vi "Main.vi"() -> ()   [LabVIEW 2010]
uses:
  GlobalVar.vi
  <vilib>/Instr/_visa.llb/VISA Configure Serial Port (Instr).vi
panel:
  out "Enum":T1(ring)
  out "error":errorcluster
  out "error Connexion":errorcluster
  out "Stop main loop":bool
  in  "stop":bool
  in  "Tab Control":T2(tab)
  out "Comm_LEDTest":bool
  out "Comm_Reception":string caption="Reception"
  in  "Comm_TestConnection":bool
  in  "baud rate":u32=9600
  in  "VISA resource name":refnum<visa-resource-name>="COM1"
  in  "timeout (10sec)":u32=10000
  out "Erreur courant":bool
  in  "Intensity (A)":string[][](array[string])
  in  "Motor right Torque (N.m)":string[][](array[string])
  out "Motor left Torque (N.m)":string[][](array[string])
  out "Batterie":string[][](array[string])
  out "Guidon":string[][](array[string])
  out "Gyroscope":string[][](array[string])
  out "AccZ":string[][](array[string])
  out "AccX":string[][](array[string])
  out "Acceleration":string[][](array[string])
  out "Velocity motor right":string[][](array[string])
  out "Velocity motor left":string[][](array[string])
  out "Angle Out of range":string[][](array[string])
  out "Speed saturation":string[][](array[string])
  out "Distance parcourue":string[][](array[string])
  out "Angle":string[][](array[string])
  out "XY Graph 2":cluster{dbl, dbl}[](graph)
  out "XY Graph":cluster{dbl, dbl}[](graph)
  in  "Time 3":dbl
  in  "Time 2":dbl
  in  "Time":dbl
  in  "Frequency 3":dbl
  out "Combo Box 3":string(combo)
  in  "Frequency 2":dbl
  out "Combo Box 2":string(combo)
  in  "Ana_SendAnalysis":bool
  in  "Frequency":dbl
  in  "Combo Box":string(combo)
  out "XY Graph 3":cluster{dbl, dbl}[](graph)
  in  "VelocitySaturation":dbl
  in  "Set velocity saturation":bool
  out "Chaîne 2":string
  out "Chaîne":string
  in  "Ready ?":bool
  in  "Current state ?":bool
  in  "Re Start system":bool
  in  "STOP system":bool
  out "tCoef Kalman":dbl
  in  "Bouton OK 11":bool
  in  "Bouton OK 10":bool
  in  "Coef Kalman":dbl
  in  "Bouton OK 9":bool
  in  "Coef System Acc":dbl
  out "tCoef DIR":dbl
  in  "Bouton OK 8":bool
  in  "Coef DIR":dbl
  in  "Bouton OK 7":bool
  out "tD":dbl
  out "tI":dbl
  out "tK":dbl
  in  "Bouton OK 6":bool
  in  "Bouton OK 5":bool
  in  "Bouton OK 4":bool
  in  "Bouton OK 3":bool
  in  "Bouton OK 2":bool
  in  "Bouton OK":bool
  in  "D":dbl
  in  "I":dbl
  in  "K":dbl
  in  "OK Button":bool
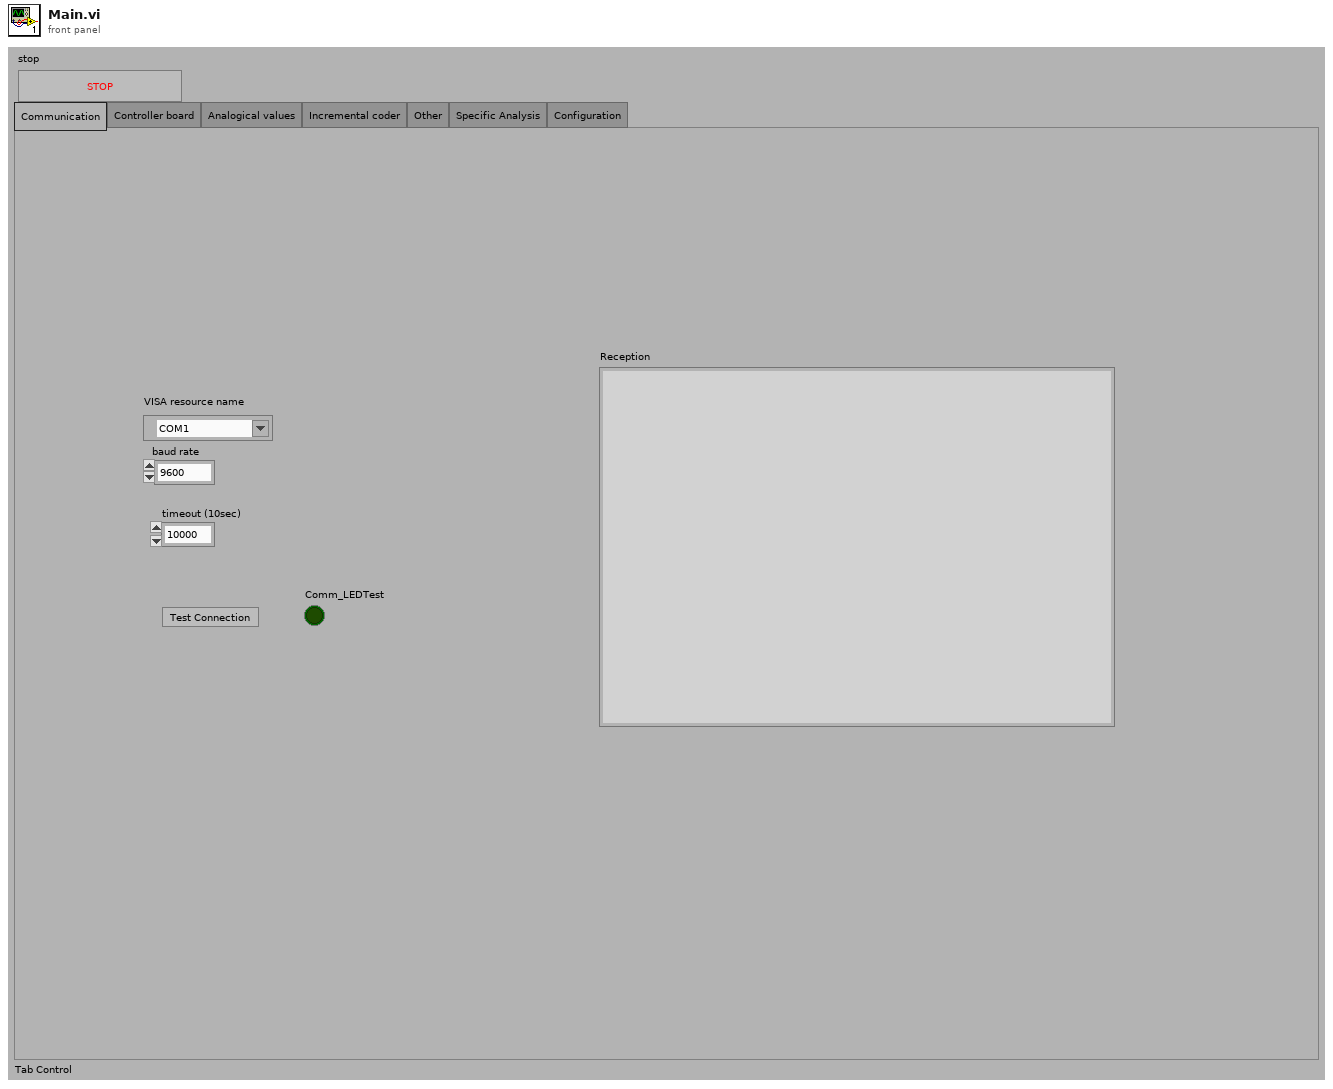
[diagram p1: front panel]
types:
  T1 = enum16{"SendAnalysis", "TestConnection", "Waiting"}
  T2 = enum32{"Communication", "Controller board", "Analogical values", "Incremental coder", "Other", "Specific Analysis", "Configuration"}
  T3 = enum8{"Enabled", "Disabled", "Disabled and Grayed Out"}
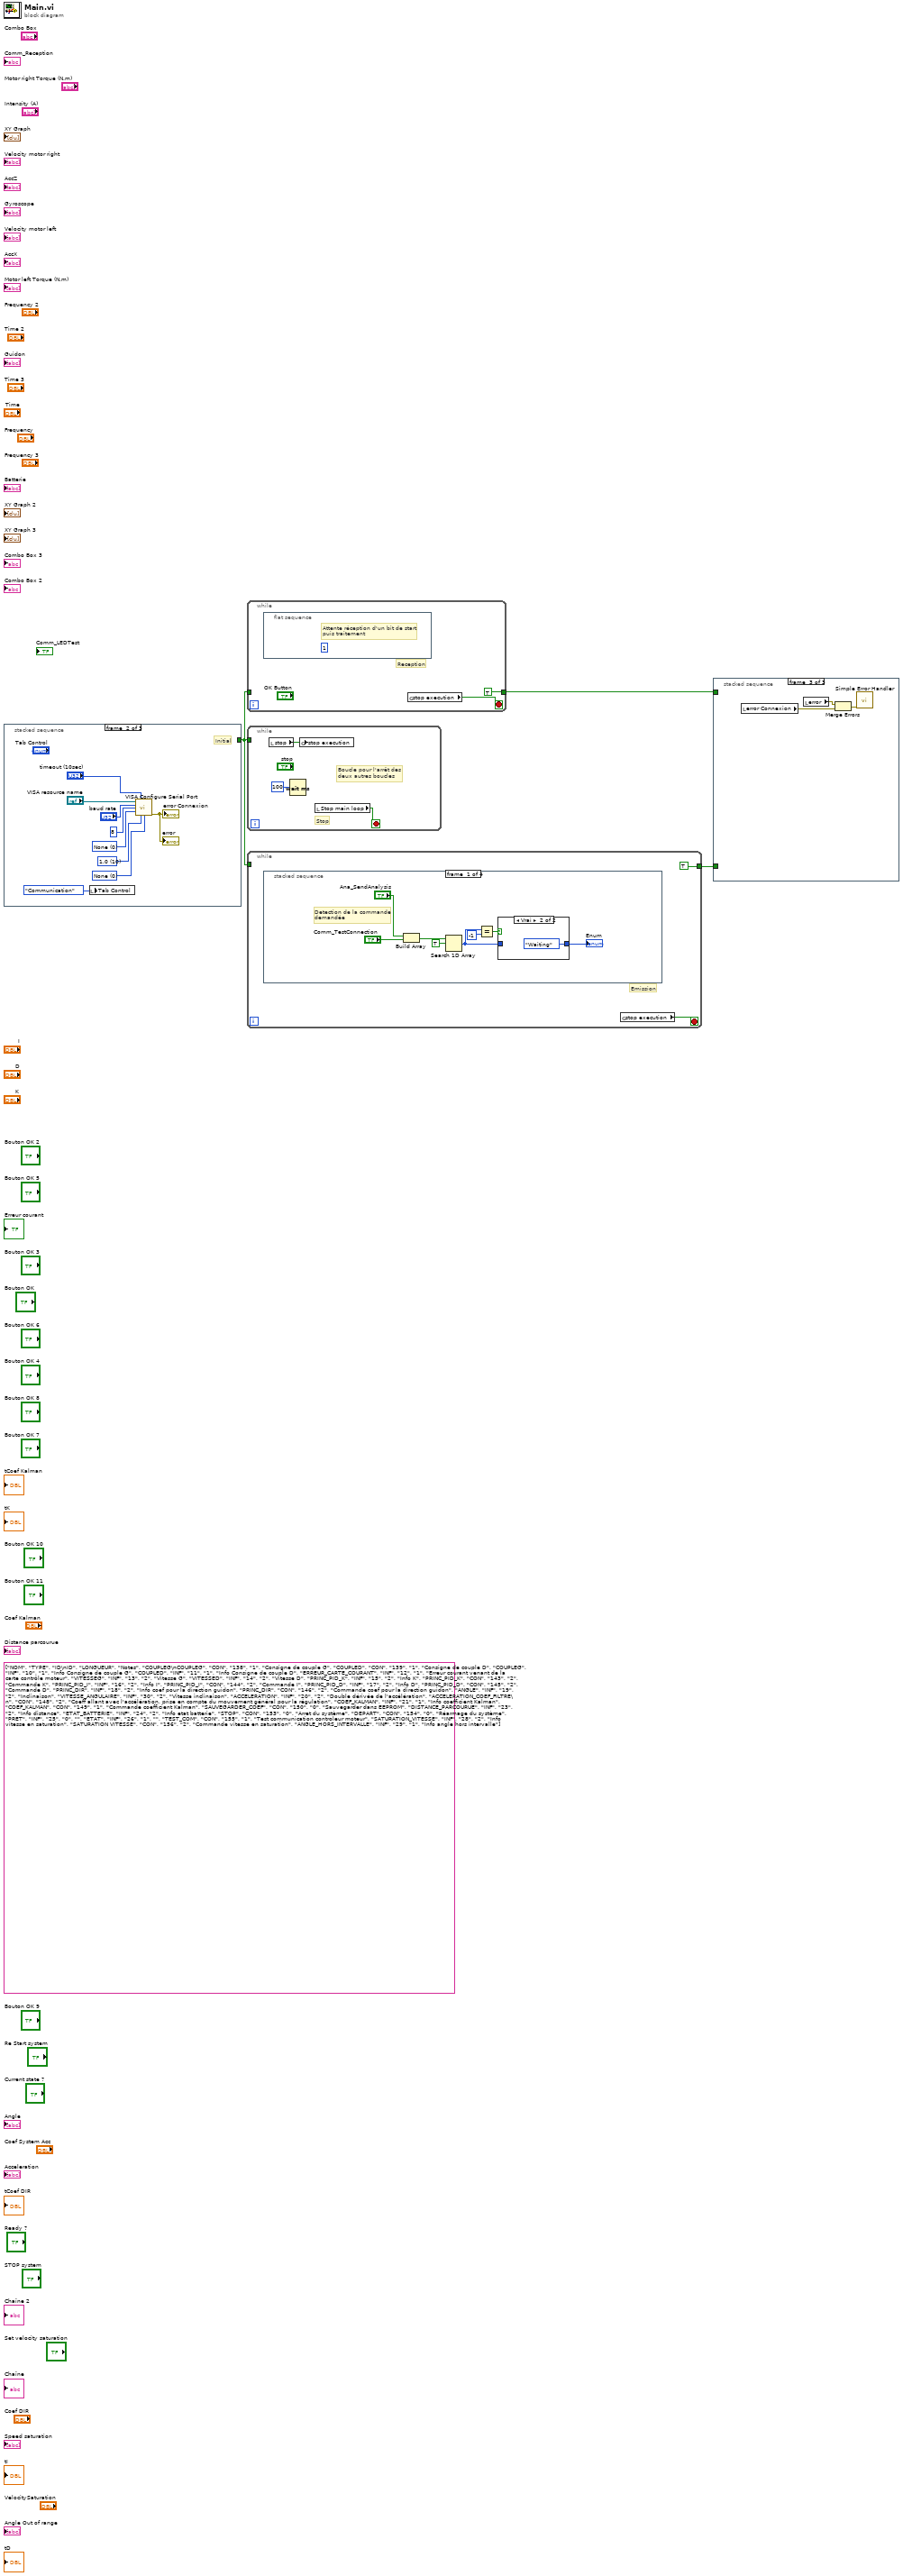
[diagram p0: block diagram]
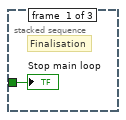
[diagram p2: hidden frame]
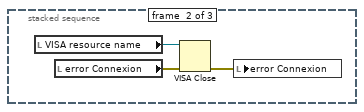
[diagram p3: hidden frame]
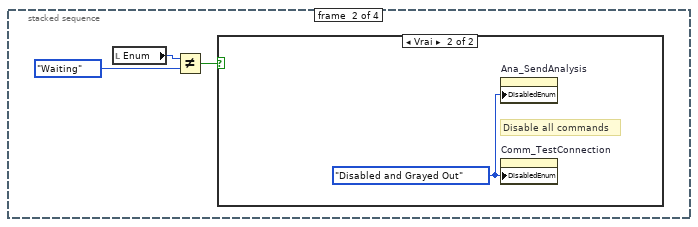
[diagram p5: hidden frame]
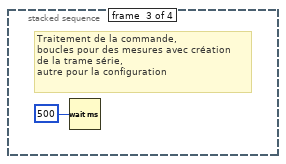
[diagram p7: hidden frame]
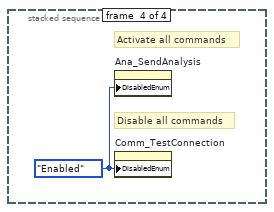
[diagram p8: hidden frame]
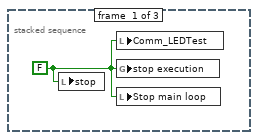
[diagram p9: hidden frame]
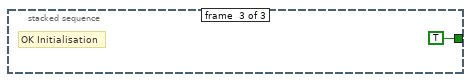
[diagram p10: hidden frame]
diagram:
  (unwired) string[][] [["NOM", "TYPE", "ID\nID", "LONGUEUR", "Notes"], ["COUPLEG\nCOUPLEG", "CON", "138", "1", "Consigne de couple G"], ["COUPLED", "CON", "139", "1", "Consigne de couple D"], ["COUPLEG", "INF", "10", "1", "Info Consigne de couple G"], ["COUPLED", "INF", "11", "1", "Info Consigne de couple D"], ["ERREUR_CARTE_COURANT", "INF", "12", "1", "Erreur courant venant de la carte contrôle moteur"], ["VITESSEG", "INF", "13", "2", "Vitesse G"], ["VITESSED", "INF", "14", "2", "Vitesse D"], ["PRINC_PID_K", "INF", "15", "2", "Info K"], ["PRINC_PID_K", "CON", "143", "2", "Commande K"], ["PRINC_PID_I", "INF", "16", "2", "Info I"], ["PRINC_PID_I", "CON", "144", "2", "Commande I"], ["PRINC_PID_D", "INF", "17", "2", "Info D"], ["PRINC_PID_D", "CON", "145", "2", "Commande D"], ["PRINC_DIR", "INF", "18", "2", "Info coef pour la direction guidon"], ["PRINC_DIR", "CON", "146", "2", "Commande coef pour la direction guidon"], ["ANGLE", "INF", "19", "2", "Inclinaison"], ["VITESSE_ANGULAIRE", "INF", "30", "2", "Vitesse inclinaison"], ["ACCELERATION", "INF", "20", "2", "Double dérivée de l'accélération"], ["ACCELERATION_COEF_FILTRE\n", "CON", "148", "2", "Coeff allant avec l'accélération, prise en compte du mouvement général pour la régulation"], ["COEF_KALMAN", "INF", "21", "1", "Info coefficient Kalman"], ["COEF_KALMAN", "CON", "149", "1", "Commande coefficient Kalman"], ["SAUVEGARDER_COEF", "CON", "150", "0", "Sauvegarder dans EEPROM"], ["DISTANCE_PARCOURUE", "INF", "23", "2", "Info distance"], ["ETAT_BATTERIE", "INF", "24", "2", "Info etat batterie"], ["STOP", "CON", "153", "0", "Arret du système"], ["DEPART", "CON", "154", "0", "Réarmage du système"], ["PRET", "INF", "25", "0", ""], ["ETAT", "INF", "26", "1", ""], ["TEST_COM", "CON", "155", "1", "Test communication controleur moteur"], ["SATURATION_VITESSE", "INF", "28", "2", "Info vitesse en saturation"], ["SATURATION VITESSE", "CON", "156", "2", "Commande vitesse en saturation"], ["ANGLE_HORS_INTERVALLE", "INF", "29", "1", "Info angle hors intervalle"]]
  n1 = stacked-sequence {
    tunnel: [_ _ TRUE] -> w3
    frame #0 {
      w4 = FALSE ("Comm_LEDTest")
      n2 = local write "stop"(w4) -> ()
      n3 = local write "Comm_LEDTest"(w4) -> ()
      n4 = global write "GlobalVar.vi" "stop execution"(w4) -> ()
      n5 = local write "Stop main loop"(w4) -> ()
    }
    frame #1 {
      w8 = u16 0 items=["None"=0, "XON/XOFF"=1, "RTS/CTS"=2, "DTR/DSR"=4] ("flow control")
      w9 = u16 10 items=["1.0"=10, "1.5"=15, "2.0"=20] ("stop bits")
      w11 = u16 0 items=["None", "Odd", "Even", "Mark", "Space"] ("parity")
      # "Initial"
      n6 = local write "Tab Control"(T2."Communication" ("Tab Control")) -> ()
      n7 = call-poly "VISA Configure Serial Port"("VISA resource name"="VISA resource name", "timeout (10sec)"="timeout (10sec)", "baud rate (9600)"="baud rate", "data bits (8)"=u16 8 ("data bits"), "parity (0:none)"=w11, "stop bits (10: 1 bit)"=w9, "flow control (0:none)"=w8) -> ("error out"=→"error Connexion" →"error":errorcluster)  [unwired: 2 in, 6 out]
    }
    frame #2 {
      # "OK Initialisation"
    }
  }
  n8 = while {
    tunnel: w3 -> [_]
    tunnel: [TRUE] -> w2
    stop <- w15 stop-if-true
    # "Reception"
    n9 = flat-sequence {
      frame #0 {
        (unwired) u32 1 ("byte count")
        # "Attente réception d'un bit de start\npuis traitement"
      }
    }
    n10 = global read "GlobalVar.vi" "stop execution"() -> (w15:bool)
  }
  n11 = while {
    tunnel: w3 -> [_]
    stop <- w18 stop-if-true
    # "Boucle pour l'arrêt des \ndeux autres boucles"
    # "Stop"
    n12 = local read "stop"() -> (w19:bool)
    n13 = Wait (ms)(milliseconds to wait=u32 100) -> ()  [unwired: 1 out]
    n14 = global write "GlobalVar.vi" "stop execution"(w19) -> ()
    n15 = local read "Stop main loop"() -> (w18:bool)
  }
  n16 = while {
    tunnel: w3 -> [_]
    tunnel: [TRUE] -> w1
    stop <- w20 stop-if-true
    # "Emission"
    n17 = stacked-sequence {
      frame #0 {
        # "Detection de la commande\ndemandée"
        n18 = Build Array("Ana_SendAnalysis", "Comm_TestConnection") -> (w27:bool[])
        n19 = Search 1D Array(1D array=w27, element=TRUE) -> (index of element=w22:i32)  [unwired: 1 in]
        n20 = Equal?(x=w22, y=-1) -> (x = y?=w24:bool)
        n21 = case shown="Vrai" w24 {
          tunnel: [w30 T1."Waiting" ("Enum 2")] -> w23
          tunnel: w22 -> [w30 _]
          frame False {
          }
          frame True {
          }
        }
        "Enum" <- w23
      }
      frame #1 {
        n22 = local read "Enum"() -> (w33:T1)
        n23 = Not Equal?(x=w33, y=T1."Waiting") -> (x != y?=w34:bool)
        n24 = case shown="Vrai" w34 {
          frame False {
          }
          frame True {
            w35 = T3."Disabled and Grayed Out" ("Disabled")
            # "Disable all commands"
            n25 = property on="Ana_SendAnalysis" class="Bool"("DisabledEnum"=w35) -> ()  [unwired: 2 in, 2 out]
            n26 = property on="Comm_TestConnection" class="Bool"("DisabledEnum"=w35) -> ()  [unwired: 2 in, 2 out]
          }
        }
      }
      frame #2 {
        # "Traitement de la commande,\nboucles pour des mesures avec création \nde la trame série,\nautre pour la configuration"
        n27 = Wait (ms)(milliseconds to wait=u32 500) -> ()  [unwired: 1 out]
      }
      frame #3 {
        w37 = T3."Enabled" ("Disabled")
        # "Disable all commands"
        # "Activate all commands"
        n28 = property on="Ana_SendAnalysis" class="Bool"("DisabledEnum"=w37) -> ()  [unwired: 2 in, 2 out]
        n29 = property on="Comm_TestConnection" class="Bool"("DisabledEnum"=w37) -> ()  [unwired: 2 in, 2 out]
      }
    }
    n30 = global read "GlobalVar.vi" "stop execution"() -> (w20:bool)
  }
  n31 = stacked-sequence {
    tunnel: w2 -> [_ _ _]
    tunnel: w1 -> [w38 _ _]
    frame #0 {
      # "Finalisation"
      "Stop main loop" <- w38
    }
    frame #1 {
      n32 = local read "VISA resource name"() -> (w41:refnum<visa-resource-name>)
      n33 = local read "error Connexion"() -> (w40:errorcluster)
      n34 = VISA Close(VISA resource name=w41, error in (no error)=w40) -> (error out=w39:errorcluster)
      n35 = local write "error Connexion"(w39) -> ()
    }
    frame #2 {
      n36 = local read "error Connexion"() -> (w44:errorcluster)
      n37 = local read "error"() -> (w43:errorcluster)
      n38 = Merge Errors(w43, w44) -> (w42:errorcluster)
      n39 = call <vilib>:"Simple Error Handler.vi"("error in (no error)"=w42) -> ()  [unwired: 4 in, 5 out]
    }
  }
